vi "S7_Write.vi"(0 "TCP":refnum<k5>, 1 "寄存器类型":u8(ring)=132 items=["I/O (P)"=128, "Input (I)"=129, "Output (Q)"=130, "Bit Memory (M)"=131, "Data (DB)"=132, "Instance Data (DI)"=133, "Local Data (L)"=134, "Predecessor Local Data (VL)"=135], 2 "DB #":u16, 5 "写入地址":u32=1, 7 "数据类型":u16(ring) items=["byte", "word", "Dword"], 9 "写入数据":u32 format="%02x", 11 "error in":errorcluster) -> (4 "TCP":refnum<k5>, 6 "写入成功":bool, 15 "error out":errorcluster)   [LabVIEW 2018]
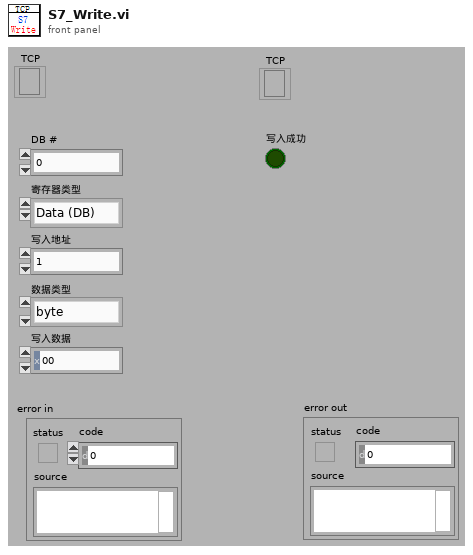
[diagram p1: front panel]
types:
  T1 = enum16{"Standard", "Buffered", "CRLF", "Immediate"}
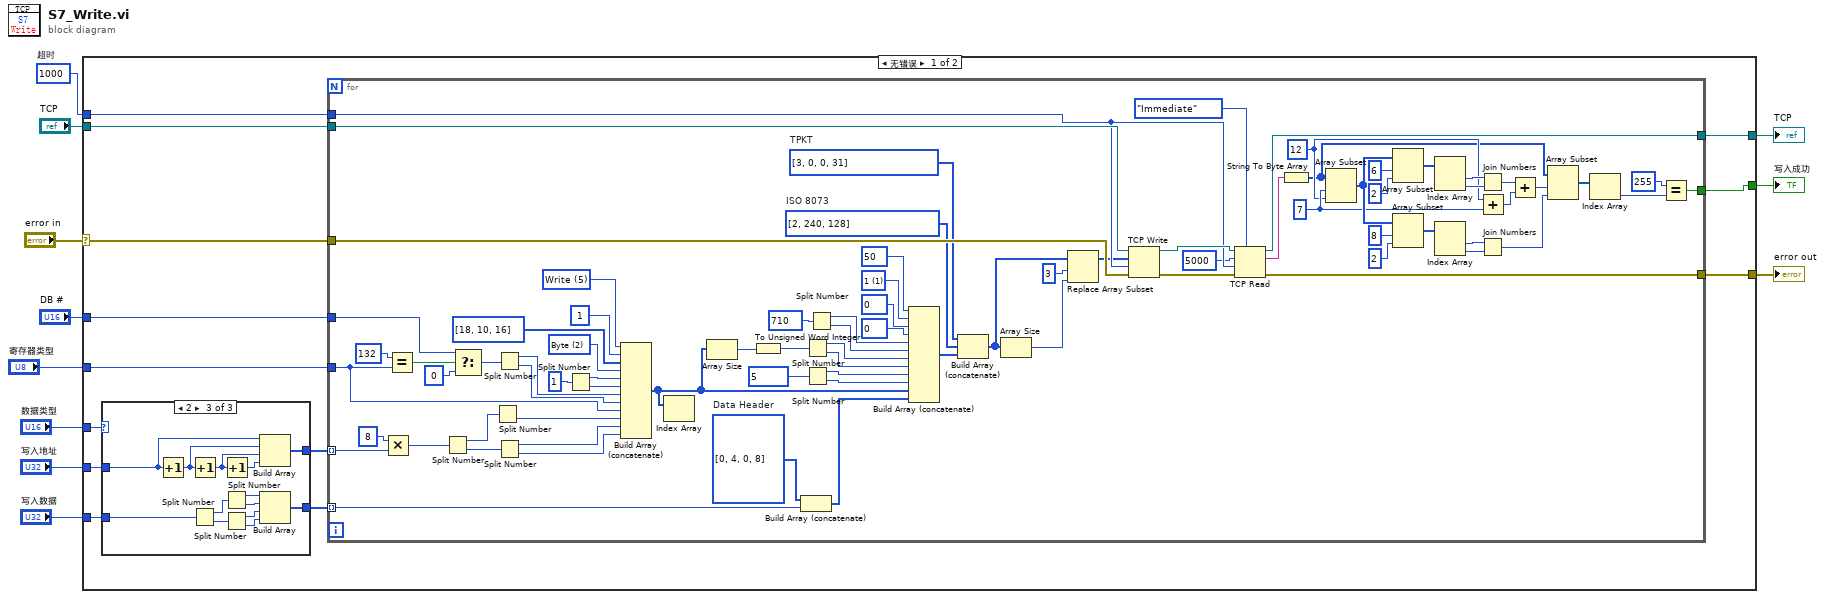
[diagram p0: block diagram]
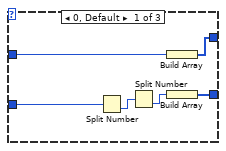
[diagram p2: hidden frame]
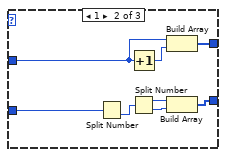
[diagram p3: hidden frame]
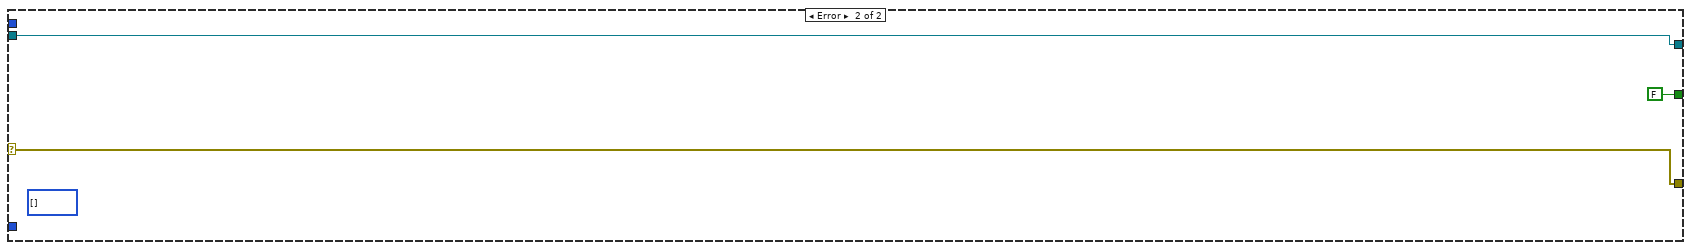
[diagram p4: hidden frame]
diagram:
  w6 = u32 1000  # 超时
  n1 = case shown="无错误" "error in" {
    selector: "error in" -> [w22 w133]
    tunnel: "TCP" -> [w23 w134]
    tunnel: w6 -> [w19 _]
    tunnel: "DB #" -> [w16 _]
    tunnel: "写入地址" -> [w14 _]
    tunnel: "寄存器类型" -> [w24 _]
    tunnel: [w21 w134] -> w7
    tunnel: [w20 w133] -> w11
    tunnel: [w12 FALSE ("Data Valid")] -> w10
    tunnel: "数据类型" -> [w15 _]
    tunnel: "写入数据" -> [w18 _]
    frame No Error {
      n2 = case shown="2" w15 {
        tunnel: w18 -> [w27 w34 w50]
        tunnel: [w30 w38 w51] -> w17
        tunnel: [w28 w36 w40] -> w13
        tunnel: w14 -> [w29 w35 w39]
        frame 0, Default {
          n3 = Split Number(x=w27) -> (lo(x)=w26:u16)  [unwired: 1 out]
          n4 = Split Number(x=w26) -> (lo(x)=w25:u8)  [unwired: 1 out]
          n5 = Build Array(w29) -> (w28:u32[])
          n6 = Build Array(w25) -> (w30:u8[])
        }
        frame 1 {
          n7 = Split Number(x=w34) -> (lo(x)=w31:u16)  [unwired: 1 out]
          n8 = Increment(x=w35) -> (x+1=w37:u32)
          n9 = Split Number(x=w31) -> (hi(x)=w33:u8, lo(x)=w32:u8)
          n10 = Build Array(w35, w37) -> (w36:u32[])
          n11 = Build Array(w33, w32) -> (w38:u8[])
        }
        frame 2 {
          n12 = Increment(x=w39) -> (x+1=w41:u32)
          n13 = Increment(x=w41) -> (x+1=w42:u32)
          n14 = Split Number(x=w50) -> (hi(x)=w49:u16, lo(x)=w48:u16)
          n15 = Increment(x=w42) -> (x+1=w43:u32)
          n16 = Split Number(x=w49) -> (hi(x)=w47:u8, lo(x)=w46:u8)
          n17 = Split Number(x=w48) -> (hi(x)=w45:u8, lo(x)=w44:u8)
          n18 = Build Array(w39, w41, w42, w43) -> (w40:u32[])
          n19 = Build Array(w47, w46, w45, w44) -> (w51:u8[])
        }
      }
      n20 = for {
        tunnel: w16 -> [w116]
        tunnel: w13 -> [w114] mode=indexing
        tunnel: w24 -> [w115]
        tunnel: w23 -> [w131]
        tunnel: w22 -> [w130]
        tunnel: [w127] -> w21
        tunnel: [w126] -> w20
        tunnel: w19 -> [w124]
        tunnel: w17 -> [w53] mode=indexing
        tunnel: [w74] -> w12
        w54 = u8[] [0, 4, 0, 8]  # Data Header
        w56 = u8[] [3, 0, 0, 31]  # TPKT
        w58 = u8[] [2, 240, 128]  # ISO 8073
        w70 = u8 1 items=["1"=1, "2"=2, "3"=3, "7"=7]
        w77 = 12 ("length")
        w78 = 7 ("index")
        w100 = u8 2 items=["Bit"=1, "Byte"=2, "Word"=4, "Dword"=6] ("Transport Type")
        w117 = u8 5 items=["Read"=4, "Write"=5] ("Read / Write")
        n21 = Multiply(x=u32 8 ("y"), y=w114) -> (x*y=w98:u32)
        n22 = Equal?(x=u8 132, y=w115) -> (x = y?=w106:bool)
        n23 = Split Number(x=w98) -> (hi(x)=w113:u16, lo(x)=w112:u16)
        n24 = Select(t=w116, s=w106, f=u16 0 ("Sequence #")) -> (s? t:f=w101:u16)
        n25 = Split Number(x=w113) -> (lo(x)=w109:u8)  [unwired: 1 out]
        n26 = Split Number(x=w101) -> (hi(x)=w102:u8, lo(x)=w103:u8)
        n27 = Split Number(x=w112) -> (hi(x)=w108:u8, lo(x)=w107:u8)
        n28 = Split Number(x=u16 1) -> (hi(x)=w110:u8, lo(x)=w99:u8)
        n29 = Build Array (concatenate)(w117, u8 1 ("Sequence #"), u8[] [18, 10, 16] ("Msg Header"), w100, w110, w99, w102, w103, w115, w109, w108, w107) -> (w55:u8[])
        n30 = Index Array(array=w55) -> ()  [unwired: 1 in, 1 out]
        n31 = Array Size(array=w55) -> (size(s)=w61:i32)
        n32 = To Unsigned Word Integer(number=w61) -> (unsigned 16bit integer=w60:u16)
        n33 = Build Array (concatenate)(w54, w53) -> (w64:u8[])
        n34 = Split Number(x=w60) -> (hi(x)=w73:u8, lo(x)=w68:u8)
        n35 = Split Number(x=u16 5 ("DLE")) -> (hi(x)=w67:u8, lo(x)=w66:u8)
        n36 = Split Number(x=u16 710 ("DLE")) -> (hi(x)=w63:u8, lo(x)=w62:u8)
        n37 = Build Array (concatenate)(u8 50 ("DLE"), w70, u8 0 ("DLE"), u8 0 ("DLE"), w63, w62, w73, w68, w67, w66, w55, w64) -> (w57:u8[])
        n38 = Build Array (concatenate)(w56, w58, w57) -> (w52:u8[])
        n39 = Array Size(array=w52) -> (size(s)=w119:i32)
        n40 = Replace Array Subset(array=w52, new element=w119, index=3) -> (w121:u8[])
        n41 = TCP Write(connection ID=w131, data in=w121, error in (no error)=w130, 9:w124) -> (connection ID out=w129:refnum<k5>, error out=w128:errorcluster)  [unwired: 1 out]
        n42 = TCP Read(connection ID=w129, bytes to read=5000, error in (no error)=w128, 7:T1."Immediate" ("mode (standard)"), 9:w124) -> (connection ID out=w127:refnum<k5>, data out=w125:string, error out=w126:errorcluster)
        n43 = String To Byte Array(string=w125) -> (unsigned byte array=w75:u8[])
        n44 = Array Subset(array=w75, index=w78, length=w77) -> (w83:u8[])
        n45 = Array Subset(array=w83, index=6, length=2) -> (w84:u8[])
        n46 = Array Subset(array=w83, index=8, length=2) -> (w89:u8[])
        n47 = Index Array(array=w84) -> (element #1=w85:u8, element #2=w86:u8)  [unwired: 2 in]
        n48 = Index Array(array=w89) -> (element #1=w88:u8, element #2=w87:u8)  [unwired: 2 in]
        n49 = Join Numbers(hi=w85, lo=w86) -> ((hi.lo)=w90:u16)
        n50 = Add(x=w77, y=w78) -> (x+y=w76:i32)
        n51 = Join Numbers(hi=w88, lo=w87) -> ((hi.lo)=w95:u16)
        n52 = Add(x=w90, y=w76) -> (x+y=w93:i32)
        n53 = Array Subset(array=w75, index=w93, length=w95) -> (w94:u8[])
        n54 = Index Array(array=w94) -> (element=w92:u8)  [unwired: 1 in]
        n55 = Equal?(x=u8 255, y=w92) -> (x = y?=w74:bool)
      }
    }
    frame Error {
      (unwired) u8[] [] ("f")
    }
  }
  "error out" <- w11
  "写入成功" <- w10
  "TCP" <- w7
